vi "Get VI Reference.vi"(8 "error in":errorcluster, 11 "id":string) -> (0 "error out":errorcluster, 3 "vi reference":refnum<vi>)   [LabVIEW 2020, in "G-AI Core.lvlib"]
uses:
  G-AI Core.lvlib
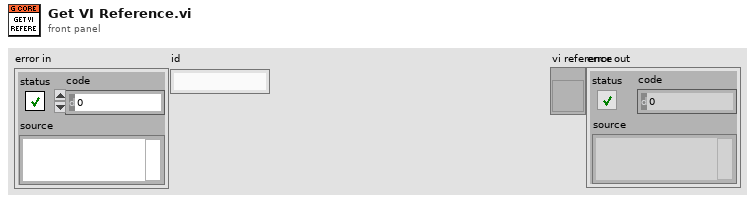
[diagram p1: front panel]
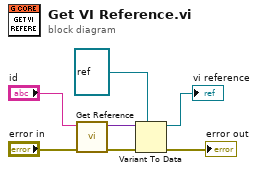
[diagram p0: block diagram]
diagram:
  n1 = call "Get Reference.vi"("error in"="error in", "id"="id") -> ("error out"=w5:errorcluster, "reference"=w6:variant)  [unwired: 8 in]
  n2 = Variant To Data(error in=w5, type=refnum<vi> refnum ("vi reference"), Variant=w6) -> (data=→"vi reference":refnum<vi>, error out=→"error out":errorcluster)
